vi "Set Error if Not Development System.vi"(8 "error in (no error)":errorcluster) -> (0 "error out":errorcluster)   [LabVIEW 2019, in "ProjectBuilder.lvlib" / "Project Builder.lvclass"]
doc: "Return an error if not called from the development system."
uses:
  Project Builder.lvclass
  <vilib>/Utility/error.llb/Error Cluster From Error Code.vi
  <vilib>/ErrorRing/Error Ring.xnode
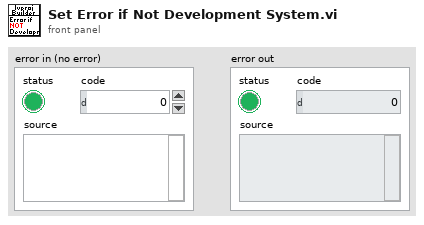
[diagram p1: front panel]
types:
  T1 = enum32{"invalid app kind", "Development System", "Run Time System", "Student Edition", "Embedded LabVIEW", "Evaluation", "Custom"}
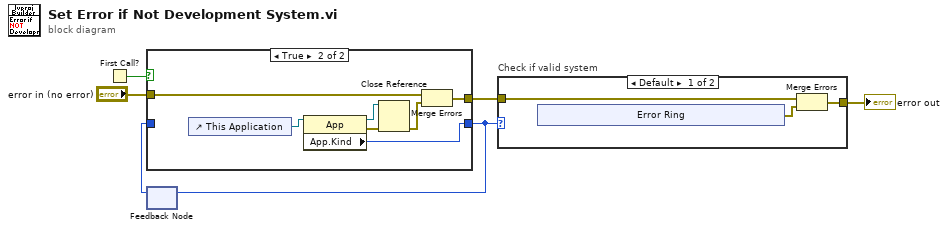
[diagram p0: block diagram]
diagram:
  n1 = First Call?() -> (First Call?: T/F=w5:bool)
  n2 = feedback #1() -> (w3:T1)  [unwired: 1 in]
  n3 = case shown="True" w5 {
    tunnel: [w7 w9] -> w1
    tunnel: [w8 w15] -> w4
    tunnel: w3 -> [w8 _]
    tunnel: "error in (no error)" -> [w7 w11]
    frame False {
    }
    frame True {
      n4 = control-ref of="This Application"() -> (w12:refnum<vi>)
      n5 = property class="App"(reference=w12) -> (reference out=w14:refnum<vi>, error out=w13:errorcluster, "App.Kind"=w15:T1)  [unwired: 1 in]
      n6 = Close Reference(reference=w14, error in (no error)=w13) -> (error out=w10:errorcluster)
      n7 = Merge Errors(w11, w10) -> (w9:errorcluster)
    }
  }
  n8 = feedback-in #1(w4) -> ()
  n9 = case "Check if valid system" shown="Default" w4 {
    tunnel: [w16 w23] -> w6
    tunnel: w1 -> [w18 w23]
    frame Default {
      n10 = xnode "Error Ring"() -> ("error out"=w17:errorcluster)
      n11 = Merge Errors(w18, w17) -> (w16:errorcluster)
    }
    frame "Development System", "Student Edition", "Evaluation" {
    }
  }
  "error out" <- w6
